vi "AngleStats_AngleMean.vi"(6 "Row":i32, 10 "Wm":T1, 11 "Sigmas":T1) -> (0 "Error":bool, 3 "Result":T1)   [LabVIEW 2019, in "Trajectory_Library.lvlib"]
doc: "Computes the mean of sigmas with the weights Wm while computing a special angle mean for a select row.\n \n\nInputs:\n - sigmas -- Sigma points.\n - Wm -- Weights for the mean.\n - Row -- The row containing the angles.\n\nOutputs:\n - Result -- Mean of sigma points."
uses:
  Trajectory_Library.lvlib
  <vilib>/Analysis/Matrix/Datatypes/RealMatrix.ctl
  <vilib>/Analysis/baseanly.llb/Real A x B.vi
  <vilib>/Analysis/NI_AALBase.lvlib
  <vilib>/Analysis/Matrix/NI_Matrix.lvlib
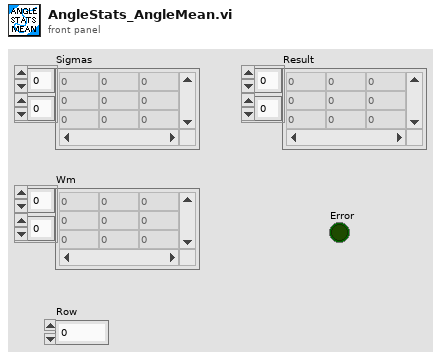
[diagram p1: front panel]
types:
  T1 = typedef "NI_Matrix.lvlib/RealMatrix.ctl" = dbl[][]
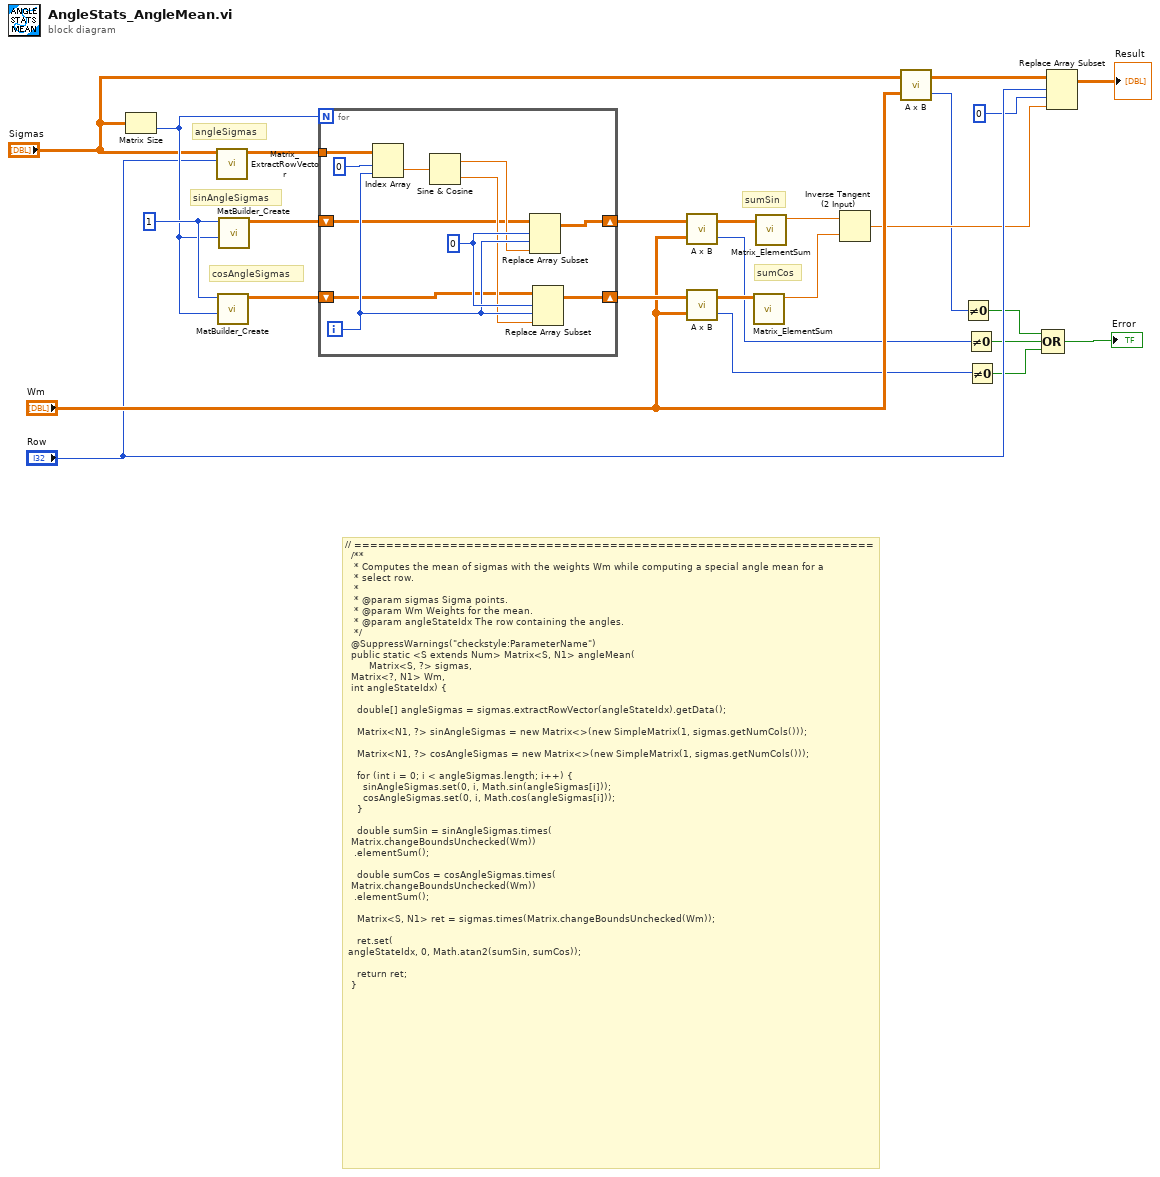
[diagram p0: block diagram]
diagram:
  w25 = 1 ("Rows")
  # "// =================================================================\n  /**\n   * Computes the mean of sigmas with the weights Wm while computing a special angle mean for a\n   * select row.\n   *\n   * @param sigmas Sigma points.\n   * @param Wm Weights for the mean.\n   * @param angleStateIdx The row containing the angles.\n   */\n  @SuppressWarnings(\"checkstyle:ParameterName\")\n  public static <S extends Num> Matrix<S, N1> angleMean(\n      \t\tMatrix<S, ?> sigmas, \n\t\tMatrix<?, N1> Wm, \n\t\tint angleStateIdx) {\n\n    double[] angleSigmas = sigmas.extractRowVector(angleStateIdx).getData();\n\n    Matrix<N1, ?> sinAngleSigmas = new Matrix<>(new SimpleMatrix(1, sigmas.getNumCols()));\n\n    Matrix<N1, ?> cosAngleSigmas = new Matrix<>(new SimpleMatrix(1, sigmas.getNumCols()));\n\n    for (int i = 0; i < angleSigmas.length; i++) {\n      sinAngleSigmas.set(0, i, Math.sin(angleSigmas[i]));\n      cosAngleSigmas.set(0, i, Math.cos(angleSigmas[i]));\n    }\n\n    double sumSin = sinAngleSigmas.times(\n\t\tMatrix.changeBoundsUnchecked(Wm))\n\t\t\t.elementSum();\n\n    double sumCos = cosAngleSigmas.times(\n\t\tMatrix.changeBoundsUnchecked(Wm))\n\t\t\t.elementSum();\n\n    Matrix<S, N1> ret = sigmas.times(Matrix.changeBoundsUnchecked(Wm));\n\n    ret.set(\n\tangleStateIdx, 0, Math.atan2(sumSin, sumCos));\n\n    return ret;\n  }"
  # "sumCos"
  # "sumSin"
  # "sinAngleSigmas"
  # "cosAngleSigmas"
  # "angleSigmas"
  n1 = Matrix Size(0:"Sigmas") -> (2:w24:i32)  [unwired: 1 out]
  n2 = call "Matrix_ExtractRowVector.vi"("Row"="Row", "input matrix"="Sigmas") -> ("output row"=w23:T1)  [unwired: 8 in, 1 out]
  n3 = call "MatBuilder_Create.vi"("Columns"=w24, "Rows"=w25) -> ("output matrix"=w21:T1)  [unwired: 9 in]
  n4 = call "MatBuilder_Create.vi"("Columns"=w24, "Rows"=w25) -> ("output matrix"=w22:T1)  [unwired: 9 in]
  n5 = for {
    N: w24 -> [_]
    tunnel: w23 -> [w36]
    shift-right: [w26] -> w20
    shift-left: w22 -> [w29]
    shift-right: [w27] -> w19
    shift-left: w21 -> [w28]
    i -> [w32]
    w33 = 0 ("disabled index (row)")
    n6 = Index Array(array=w36, index (row)=0, index (col)=w32) -> (element=w34:dbl)
    n7 = Sine & Cosine(0:w34) -> (1:w31:dbl, 2:w30:dbl)
    n8 = Replace Array Subset(array=w29, new element=w31, index (row)=w33, index (col)=w32) -> (w26:T1)
    n9 = Replace Array Subset(array=w28, new element=w30, index (row)=w33, index (col)=w32) -> (w27:T1)
  }
  n10 = call-poly <vilib>:"A x B.vi"("B"="Wm", "A"=w20) -> ("error"=w3:i32, "A x B"=w16:T1)
  n11 = call-poly <vilib>:"A x B.vi"("B"="Wm", "A"=w19) -> ("error"=w2:i32, "A x B"=w15:T1)
  n12 = call "Matrix_ElementSum.vi"("input matrix"=w15) -> ("Sum"=w13:dbl)  [unwired: 10 in]
  n13 = call "Matrix_ElementSum.vi"("input matrix"=w16) -> ("Sum"=w14:dbl)  [unwired: 10 in]
  n14 = Inverse Tangent (2 Input)(1:w13, 2:w14) -> (0:w10:dbl)
  n15 = call-poly <vilib>:"A x B.vi"("B"="Wm", "A"="Sigmas") -> ("error"=w7:i32, "A x B"=w9:T1)
  n16 = Not Equal To 0?(x=w7) -> (x != 0?=w6:bool)
  n17 = Not Equal To 0?(x=w3) -> (x != 0?=w5:bool)
  n18 = Not Equal To 0?(x=w2) -> (x != 0?=w4:bool)
  n19 = Compound Arithmetic op=OR(w6, w5, w4) -> (→"Error":bool)
  n20 = Replace Array Subset(array=w9, new element=w10, index (row)="Row", index (col)=0 ("disabled index (col)")) -> (→"Result":T1)
